vi "Scroll Watcher.vi"(0 "Exit Command":refnum<user-event>, 5 "NewVal":refnum<user-event>) -> ()   [LabVIEW 2015, in "QuickVIew.lvlib"]
doc: "TLB Prime - Application Template 1.3.0.24\nNorm Kirchner, NI Systems Engineering - NI\nCopyright (c) 2014, NI"
uses:
  QuickVIew.lvlib
  <vilib>/Utility/inputDevices.llb/keyboardAcquire.vi
  <vilib>/Utility/inputDevices.llb/mouseAcquire.vi
  <vilib>/Utility/inputDevices.llb/closeMouse.vi
  Dependencies.llb/TLB`_Dependencies.lvlib
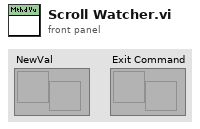
[diagram p1: front panel]
types:
  T1 = enum16{"0", "1", "2", "3", "4", "5", "6", "7", "8", "9", "A", "B", "C", "D", "E", "F", "G", "H", "I", "J", "K", "L", "M", "N", "O", "P", "Q", "R", "S", "T", "U", "V", "W", "X", "Y", "Z", "F1", "F2", "F3", "F4", "F5", "F6", "F7", "F8", "F9", "F10", "F11", "F12", "F13", "F14", "F15", "ADD", "BACK", "BACKSLASH", "CAPITAL", "COMMA", "DECIMAL", "DELETE", "DIVIDE", "DOWN", "END", "EQUALS", "ESCAPE", "GRAVE (`)", "HOME", "INSERT", "LBRACKET", "LCONTROL", "LEFT", "L ALT", "LSHIFT", "LWIN", "MINUS", "MULTIPLY", "NEXT", "NUMLOCK", "NUMPAD_0", "NUMPAD_1", "NUMPAD_2", "NUMPAD_3", "NUMPAD_4", "NUMPAD_5", "NUMPAD_6", "NUMPAD_7", "NUMPAD_8", "NUMPAD_9", "PAUSE", "PERIOD", "PRIOR (PG UP)", "RBRACKET", "RCONTROL", "RETURN", "RIGHT", "R ALT", "RSHIFT", "RWIN", "SCROLL", "SEMICOLON", "SLASH", "SPACE", "SUBTRACT", "TAB", "UP", "ENTER (num pad)", "' (quote)"}
  T2 = cluster{"Horizontal":i32, "Vertical":i32, "Scrolling":i32}
  T3 = enum16{"0", "1", "2", "3", "4", "5", "6", "7", "8", "9", "A", "B", "C", "D", "E", "F", "G", "H", "I", "J", "K", "L", "M", "N", "O", "P", "Q", "R", "S", "T", "U", "V", "W", "X", "Y", "Z", "F1", "F2", "F3", "F4", "F5", "F6", "F7", "F8", "F9", "F10", "F11", "F12", "F13", "F14", "F15", "ADD", "BACK", "BACKSLASH", "CAPITAL", "COMMA", "DECIMAL", "DELETE", "DIVIDE", "DOWN", "END", "EQUALS", "ESCAPE", "GRAVE (`)", "HOME", "INSERT", "LBRACKET", "LCONTROL", "LEFT", "L ALT", "LSHIFT", "LWIN", "MINUS", "MULTIPLY", "NEXT", "NUMLOCK", "NUMPAD_0", "NUMPAD_1", "NUMPAD_2", "NUMPAD_3", "NUMPAD_4", "NUMPAD_5", "NUMPAD_6", "NUMPAD_7", "NUMPAD_8", "NUMPAD_9", "PAUSE", "PERIOD", "PRIOR (PG UP)", "RBRACKET", "RCONTROL", "RETURN", "RIGHT", "R ALT", "RSHIFT", "RWIN", "SCROLL", "SEMICOLON", "SLASH", "SPACE", "SUBTRACT", "TAB", "UP", "ENTER (num pad)", "' (quote)"}[]
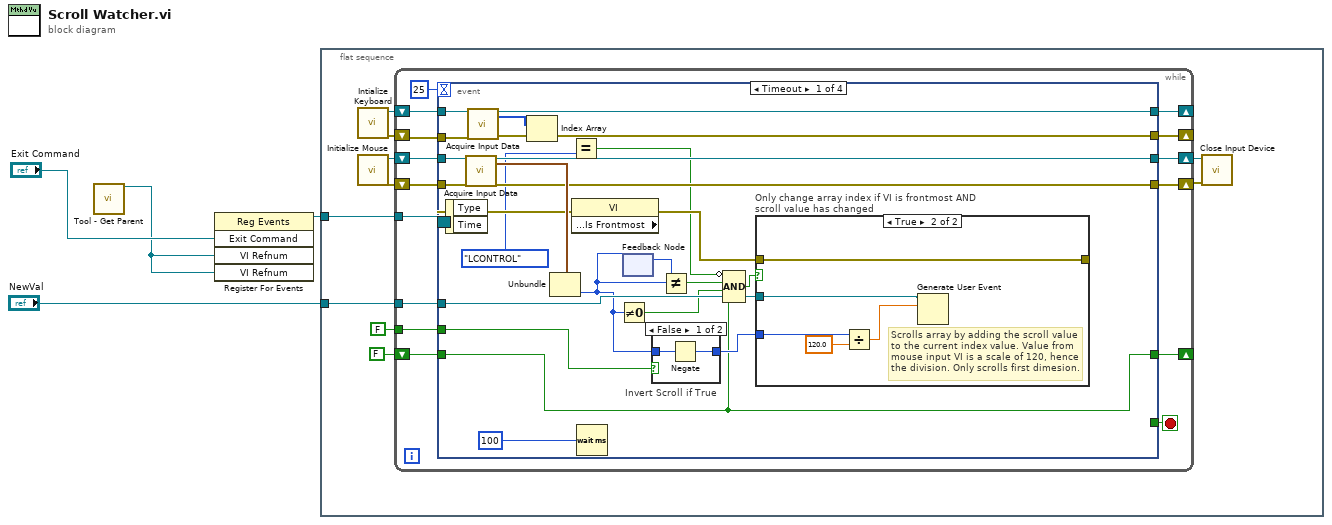
[diagram p0: block diagram]
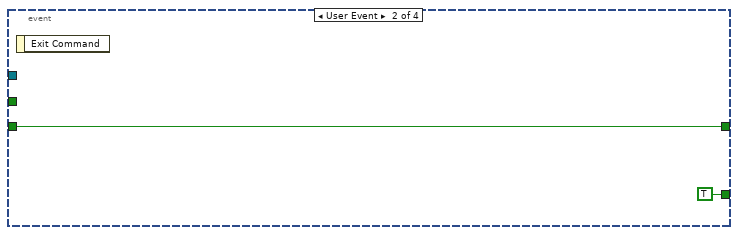
[diagram p4: hidden frame]
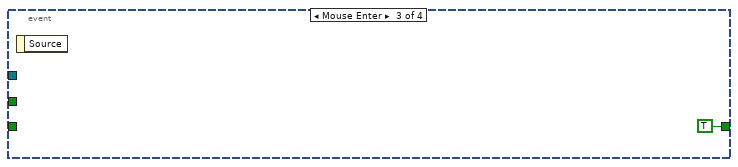
[diagram p5: hidden frame]
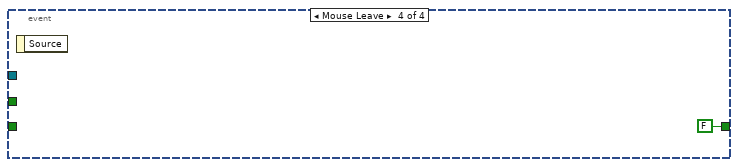
[diagram p6: hidden frame]
diagram:
  n1 = call "Tool - Get Parent.vi"() -> ("VI Refnum"=w1:refnum<vi>)  [unwired: 17 in, 2 out]
  n2 = register-events("Exit Command", w1, w1) -> (reference out=w3:refnum<event-registration>)  [unwired: 2 in, 1 out]
  n3 = flat-sequence {
    tunnel: "NewVal" -> [w9]
    tunnel: w3 -> [w8]
    frame #0 {
      n4 = call <vilib>:"Intialize Keyboard.vi"() -> ("error out"=w5:errorcluster, "device ID"=w6:refnum<k1>)  [unwired: 10 in]
      n5 = call <vilib>:"Initialize Mouse.vi"() -> ("error out"=w10:errorcluster, "device ID"=w11:refnum<k1>)  [unwired: 10 in]
      n6 = while {
        shift-right: [w26] -> w14
        shift-left: w11 -> [w28]
        shift-right: [w24] -> w13
        shift-left: w10 -> [w25]
        tunnel: FALSE ("Invert Scroll (false)") -> [w27]
        tunnel: w9 -> [w22]
        tunnel: w8 -> [w21]
        shift-right: [w19] -> _
        shift-left: FALSE ("Invert Scroll (false)") -> [w20]
        shift-right: [w15] -> _
        shift-left: w5 -> [w17]
        shift-right: [w16] -> _
        shift-left: w6 -> [w18]
        stop <- w29 stop-if-true
        n7 = event shown="[0] Timeout" {
          selector: w21 -> [_ _ _ _]
          dyn-events: _ -> [_ _ _ _]
          timeout: 25 -> [_ _ _ _]
          tunnel: [_ TRUE ("Stop") _ _] -> w29
          tunnel: w28 -> [w51 _ _ _]
          tunnel: w27 -> [w49 _ _ _]
          tunnel: [w48 _ _ _] -> w26
          tunnel: w25 -> [w44 _ _ _]
          tunnel: [w43 _ _ _] -> w24
          tunnel: w22 -> [w53 _ _ _]
          tunnel: w20 -> [w31 w63 _ _]
          tunnel: [w31 w63 TRUE ("Invert Scroll (false)") FALSE ("Invert Scroll (false)")] -> w19
          tunnel: w18 -> [w42 _ _ _]
          tunnel: w17 -> [w41 _ _ _]
          tunnel: [w40 _ _ _] -> w16
          tunnel: [w39 _ _ _] -> w15
          event Timeout {
            n8 = event-data() -> ()  [unwired: 1 in, 2 out]
            n9 = call-poly <vilib>:"Acquire Input Data.vi"("device ID"=w51, "error in (no error)"=w44) -> ("device ID"=w48:refnum<k1>, "axis info"=w45:T2, "error out"=w43:errorcluster)  [unwired: 14 in, 1 out]
            n10 = call-poly <vilib>:"Acquire Input Data.vi"("device ID"=w42, "error in (no error)"=w41) -> ("device ID"=w40:refnum<k1>, "keys pressed"=w38:T3, "error out"=w39:errorcluster)  [unwired: 15 in]
            n11 = Index Array(array=w38) -> (element=w37:T1)  [unwired: 1 in]
            n12 = Unbundle(w45) -> ("Scrolling"=w30:i32)  [unwired: 2 out]
            n13 = Equal?(x=w37, y=T1."LCONTROL" ("element")) -> (x = y?=w35:bool)
            n14 = property class="VI" props=["Front Panel Window:Is Frontmost"](error in=w44) -> (error out=w46:errorcluster)  [unwired: 1 in, 2 out]
            n15 = Wait (ms)(milliseconds to wait=u32 100) -> ()  [unwired: 1 out]
            n16 = Not Equal To 0?(x=w30) -> (x != 0?=w32:bool)
            n17 = feedback-in #1(w30) -> ()
            n18 = feedback #1() -> (w33:i32)  [unwired: 1 in]
            n19 = case "Invert Scroll if True" shown="False" w49 {
              tunnel: [w54 w56] -> w47
              tunnel: w30 -> [w55 w56]
              frame False {
                n20 = Negate(x=w55) -> (-x=w54:i32)
              }
              frame True {
              }
            }
            n21 = Not Equal?(x=w33, y=w30) -> (x != y?=w34:bool)
            n22 = Compound Arithmetic op=AND(invert w35, w34, w32, w31) -> (w50:bool)
            n23 = case "Only change array index if VI is frontmost AND scroll value has changed" shown="True" w50 {
              tunnel: w47 -> [_ w62]
              tunnel: [w57 w58] -> _
              tunnel: w46 -> [w57 w58]
              tunnel: w53 -> [_ w60]
              frame False {
              }
              frame True {
                # "Scrolls array by adding the scroll value to the current index value. Value from mouse input VI is a scale of 120, hence the division. Only scrolls first dimesion."
                n24 = Divide(x=w62, y=sgl 120.0) -> (x/y=w59:sgl)
                n25 = Generate User Event(user event=w60, event data cluster=w59) -> ()  [unwired: 2 in, 2 out]
              }
            }
          }
          event User Event {
            n26 = event-data() -> ()  [unwired: 1 in, 1 out]
          }
          event Mouse Enter {
            n27 = event-data() -> ()  [unwired: 1 in, 1 out]
          }
          event Mouse Leave {
            n28 = event-data() -> ()  [unwired: 1 in, 1 out]
          }
        }
      }
      n29 = call-poly <vilib>:"Close Input Device.vi"("error in (no error)"=w13, "device ID"=w14) -> ()  [unwired: 8 in, 1 out]
    }
  }
